vi "Read Log.vi"(11 "Log in":refnum<class "Log.lvclass">) -> (2 "Log":T1={"Log Directory"=path "", "Log Filename Base"="", "Max records per file"=1000, "Comment"=""} {"Max records per file" min=100 max=1000000}, 3 "Log out":refnum<class "Log.lvclass">)   [LabVIEW 2013, in "Log.lvclass"]
uses:
  Log.lvclass
  Configuration/Log.ctl
  Log.lvclass/Log.ctl
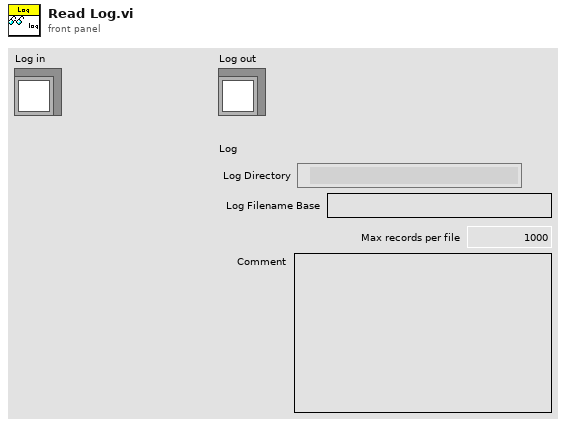
[diagram p1: front panel]
types:
  T1 = typedef "Log.ctl" = cluster{"Log Directory":path, "Log Filename Base":string, "Max records per file":u32, "Comment":string}
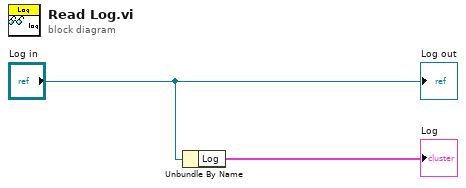
[diagram p0: block diagram]
diagram:
  n1 = Unbundle By Name("Log in") -> ("Log"=→"Log":T1)
  "Log out" <- "Log in"
